vi "Read UI Constants.vi"(8 "error in (no error)":errorcluster, 11 "CFG File Refnum in":T2) -> (0 "error out":errorcluster, 2 "MHL Configuration":T1, 3 "CFG File Refnum out":T2)   [LabVIEW 2015]
uses:
  <vilib>/Utility/config.llb/Config Data RefNum.ctl
  controls/MHL Configuration.ctl
  support/Boiler System Globals.vi
  <vilib>/Utility/config.llb/Read Key (Double).vi
  <vilib>/Utility/config.llb/NI_LVConfig.lvlib
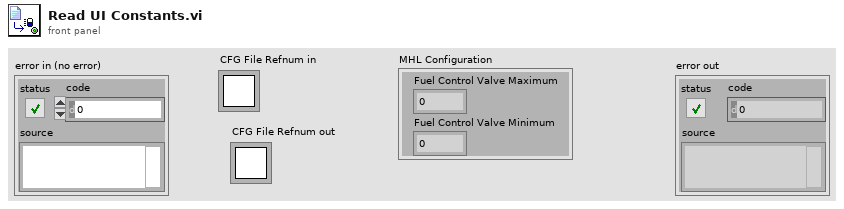
[diagram p1: front panel]
types:
  T1 = typedef "MHL Configuration.ctl" = cluster{"Fuel Control Valve Maximum":dbl, "Fuel Control Valve Minimum":dbl}
  T2 = typedef "NI_LVConfig.lvlib/Config Data RefNum.ctl" = refnum<k1>
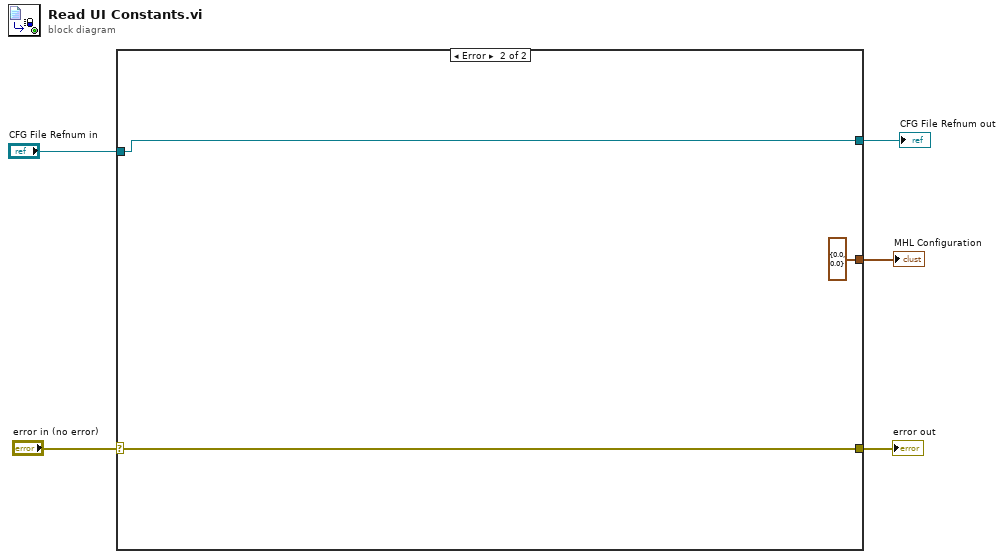
[diagram p0: block diagram]
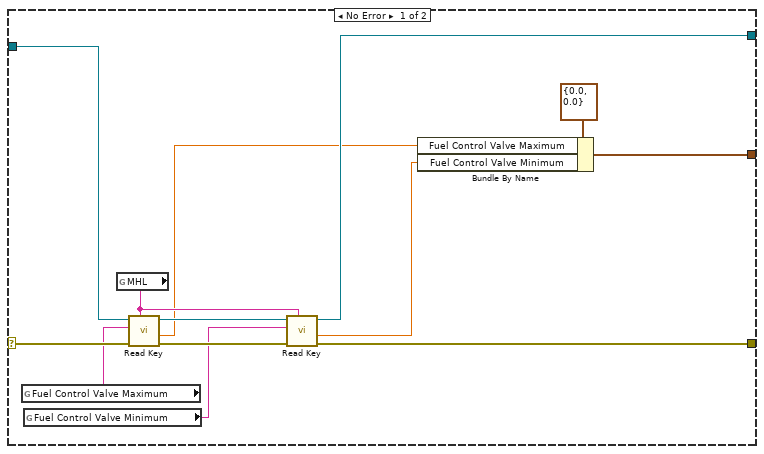
[diagram p2: hidden frame]
diagram:
  n1 = case shown="Error" "error in (no error)" {
    selector: "error in (no error)" -> [w18 w20]
    tunnel: [w16 w20] -> w4
    tunnel: "CFG File Refnum in" -> [w14 w19]
    tunnel: [w12 w19] -> w2
    tunnel: [w6 T1 {"Fuel Control Valve Maximum"=0.0, "Fuel Control Valve Minimum"=0.0} ("MHL Configuration")] -> w1
    frame No Error {
      n2 = global read "Boiler System Globals.vi" "Fuel Control Valve Maximum"() -> (w11:string)
      n3 = global read "Boiler System Globals.vi" "Fuel Control Valve Minimum"() -> (w10:string)
      n4 = global read "Boiler System Globals.vi" "MHL"() -> (w15:string)
      n5 = call-poly <vilib>:"Read Key.vi"("section"=w15, "error in (no error)"=w18, "key"=w11, "refnum"=w14) -> ("error out"=w17:errorcluster, "value"=w7:dbl, "refnum out"=w13:T2)  [unwired: 4 in, 1 out]
      n6 = call-poly <vilib>:"Read Key.vi"("section"=w15, "error in (no error)"=w17, "key"=w10, "refnum"=w13) -> ("error out"=w16:errorcluster, "value"=w8:dbl, "refnum out"=w12:T2)  [unwired: 4 in, 1 out]
      n7 = Bundle By Name(cluster=T1 {"Fuel Control Valve Maximum"=0.0, "Fuel Control Valve Minimum"=0.0} ("MHL Configuration"), "Fuel Control Valve Maximum"=w7, "Fuel Control Valve Minimum"=w8) -> (w6:T1)
    }
    frame Error {
    }
  }
  "error out" <- w4
  "CFG File Refnum out" <- w2
  "MHL Configuration" <- w1
